vi "Get Index.vi"(8 "error in":errorcluster, 11 "OD Subentry in":refnum<class "OD Subentry.lvclass">) -> (0 "error out":errorcluster, 2 "Index":u16, 3 "OD Subentry out":refnum<class "OD Subentry.lvclass">)   [LabVIEW 2024, in "OD Subentry.lvclass"]
uses:
  OD Subentry.lvclass
  OD Subentry.lvclass/OD Subentry.ctl
  OD Entry/OD Entry.lvclass
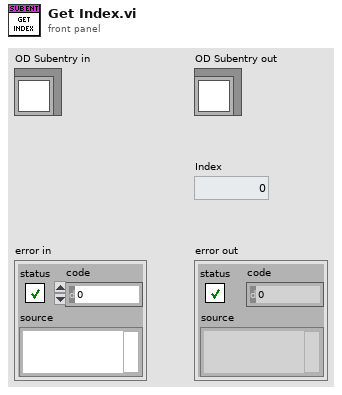
[diagram p1: front panel]
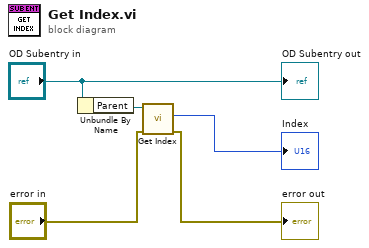
[diagram p0: block diagram]
diagram:
  n1 = Unbundle By Name("OD Subentry in") -> ("Parent"=w4:refnum<class "OD Entry.lvclass">)
  n2 = call-dynamic "Get Index.vi"("error in (no error)"="error in", "OD Entry in"=w4) -> ("error out"=→"error out":errorcluster, "Index"=→"Index":u16)  [unwired: 7 in, 1 out]
  "OD Subentry out" <- "OD Subentry in"
